vi "Get_Users_IDs.vi"(8 "error in (no error)":errorcluster, 11 "DB in":refnum<class "DB.lvclass">) -> (0 "error out":errorcluster, 1 "Project_ID_arr":string="0", 2 "User_ID":i16, 3 "DB out":refnum<class "DB.lvclass">)   [LabVIEW 2020, in "DB.lvclass"]
uses:
  DB.lvclass
  DB.lvclass/DB.ctl
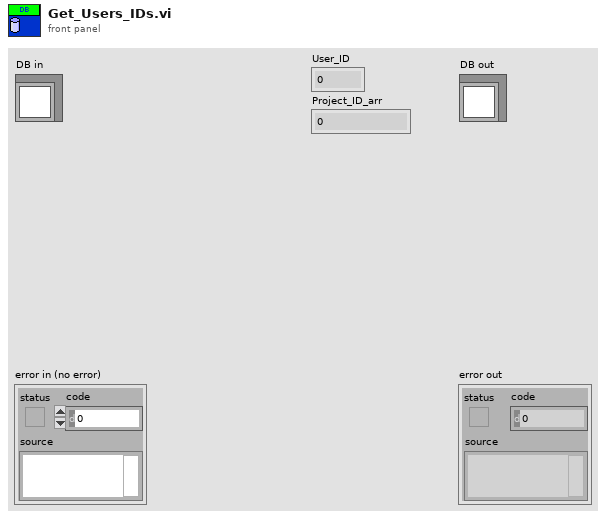
[diagram p1: front panel]
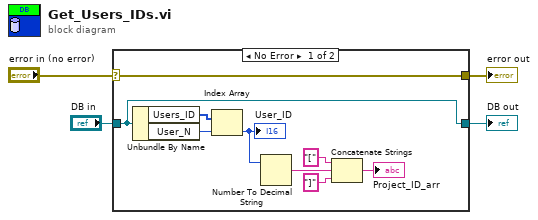
[diagram p0: block diagram]
diagram:
  n1 = case shown="No Error" "error in (no error)" {
    selector: "error in (no error)" -> [w13 w15]
    tunnel: [w13 w15] -> w3
    tunnel: [w12 w14] -> w1
    tunnel: "DB in" -> [w12 w14]
    frame No Error {
      n2 = Unbundle By Name(w12) -> ("Users_ID"=w11:i16[], "User_N"=w10:i16)
      n3 = Index Array(array=w11, index=w10) -> (element=w9:i16)
      "User_ID" <- w9
      n4 = Number To Decimal String(number=w9) -> (decimal integer string=w7:string)  [unwired: 1 in]
      n5 = Concatenate Strings("[" ("string"), w7, "]" ("string")) -> (→"Project_ID_arr":string)
    }
    frame Error {
    }
  }
  "error out" <- w3
  "DB out" <- w1
